vi "SharedVariable.Write.vi"(8 "error in":errorcluster, 9 "value":string, 10 "variable":string) -> (0 "error out":errorcluster, 1 "found":bool)   [LabVIEW 2019, in "Tools.lvlib"]
uses:
  Tools.lvlib
  ProjectPaths.vi
  <vilib>/Utility/config.llb/Write Key (String).vi
  <vilib>/Utility/config.llb/NI_LVConfig.lvlib
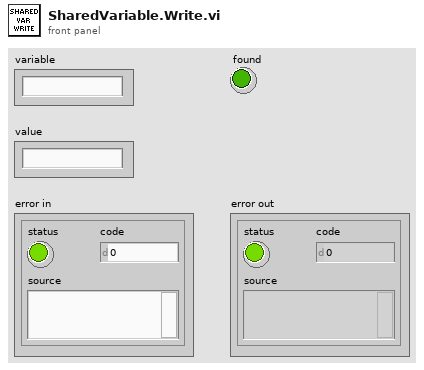
[diagram p1: front panel]
types:
  T1 = typedef "NI_LVConfig.lvlib/Config Data RefNum.ctl" = refnum<k1>
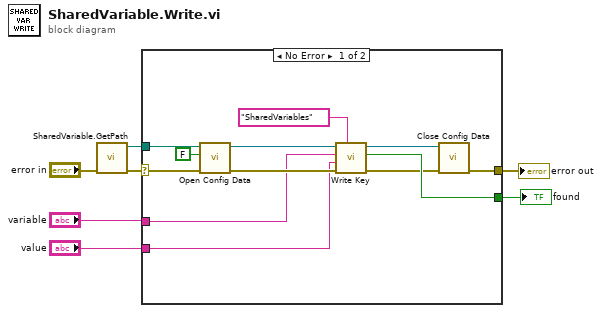
[diagram p0: block diagram]
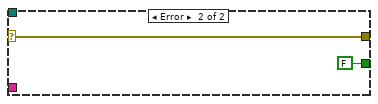
[diagram p2: hidden frame]
diagram:
  n1 = call "SharedVariable.GetPath.vi"("error in (no error)"="error in") -> ("error out"=w7:errorcluster, "Shared Variables path"=w6:path)  [unwired: 9 in]
  n2 = case shown="No Error" w7 {
    selector: w7 -> [w19 w21]
    tunnel: w6 -> [w18 _]
    tunnel: "variable" -> [w11 _]
    tunnel: "value" -> [w8 _]
    tunnel: [w13 FALSE ("found?")] -> w2
    tunnel: [w14 w21] -> w1
    frame No Error {
      n3 = call <vilib>:"Open Config Data.vi"("error in (no error)"=w19, "create file if necessary (T)"=FALSE, "configuration file path"=w18) -> ("error out"=w16:errorcluster, "refnum"=w10:T1)  [unwired: 6 in, 1 out]
      n4 = call-poly <vilib>:"Write Key.vi"("section"="SharedVariables", "error in (no error)"=w16, "value"=w8, "key"=w11, "refnum"=w10) -> ("error out"=w12:errorcluster, "found?"=w13:bool, "refnum out"=w15:T1)  [unwired: 4 in]
      n5 = call <vilib>:"Close Config Data.vi"("error in (no error)"=w12, "refnum"=w15) -> ("error out"=w14:errorcluster)  [unwired: 8 in, 1 out]
    }
    frame Error {
    }
  }
  "error out" <- w1
  "found" <- w2
